vi "TP Buffer Check Timeout on Connections.vi"(0 "Connections":T1[](array[typedef]), 7 "Time Out":u32=200, 11 "error in (no error)":errorcluster) -> (4 "Timed Out Connections?":bool, 8 "Index Array":i32[](array[numeric]), 15 "error out":errorcluster)   [LabVIEW 2013, in "J1939.lvlib"]
uses:
  J1939.lvlib
  TP Buffer Connection Cluster.ctl
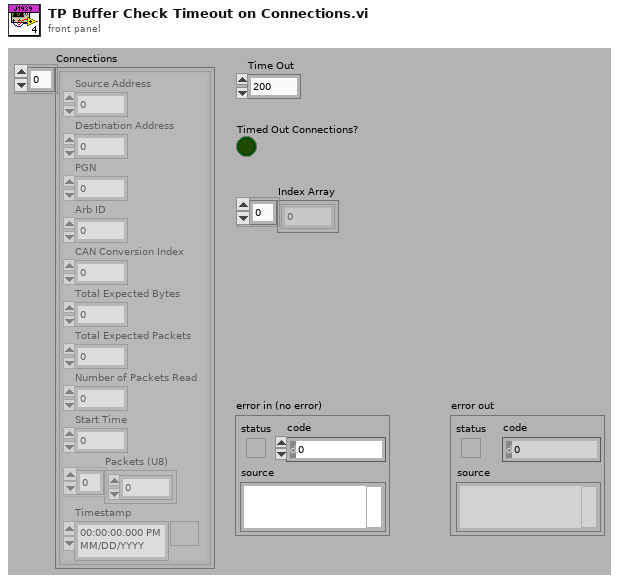
[diagram p1: front panel]
types:
  T1 = typedef "J1939.lvlib/TP Buffer Connection Cluster.ctl" = cluster{"Source Address":u8, "Destination Address":u8, "PGN":u32, "Arb ID":u32, "CAN Conversion Index":u32, "Total Expected Bytes":u16, "Total Expected Packets":u8, "Number of Packets Read":u8, "Start Time":u32, "Packets (U8)":u8[], "Timestamp":timestamp}
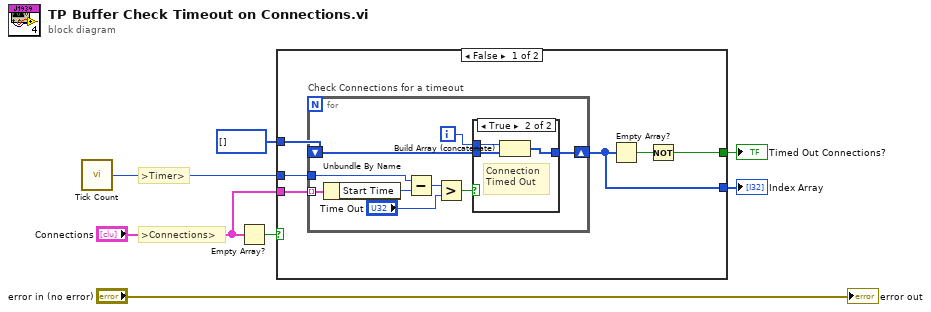
[diagram p0: block diagram]
diagram:
  # ">Timer>"
  # ">Connections>"
  n1 = call "Tick Count"() -> ("Tick Count(mSec)"=w7:u32)
  n2 = Empty Array?(array="Connections") -> (empty?=w4:bool)
  n3 = case shown="False" w4 {
    tunnel: "Connections" -> [w11 _]
    tunnel: w7 -> [w13 _]
    tunnel: i32[] [] -> [w12 _]
    tunnel: [w9 _] -> w2
    tunnel: [w8 _] -> w1
    frame False {
      n4 = for "Check Connections for a timeout" {
        tunnel: w11 -> [w22] mode=indexing
        tunnel: w13 -> [w21]
        shift-right: [w18] -> w8
        shift-left: w12 -> [w17]
        i -> [w19]
        n5 = Unbundle By Name(w22) -> ("Start Time"=w20:u32)
        n6 = Subtract(x=w21, y=w20) -> (x-y=w16:u32)
        n7 = Greater?(x=w16, y="Time Out") -> (0:w14:bool)
        n8 = case shown="True" w14 {
          tunnel: w19 -> [_ w26]
          tunnel: [w23 w25] -> w18
          tunnel: w17 -> [w23 w24]
          frame False {
          }
          frame True {
            # "Connection\nTimed Out"
            n9 = Build Array (concatenate)(w26, w24) -> (w25:i32[])
          }
        }
      }
      n10 = Empty Array?(array=w8) -> (empty?=w10:bool)
      n11 = Not(x=w10) -> (.not. x?=w9:bool)
    }
    frame True {
      # "No Connections"
    }
  }
  "Timed Out Connections?" <- w2
  "Index Array" <- w1
  "error out" <- "error in (no error)"
